vi "RW Current Limits.vi"(7 "Write?":bool, 8 "Low Lim 2":dbl[](array[numeric])=[-1.0, -1.0, -1.0, -1.0, -1.0, 3.5, 3.5, -1.0, -1.0, -1.0, -1.0, -1.0, -1.0, -1.0, -1.0, -1.0, -1.0, -1.0, -1.0, -1.0, -1.0, -1.0, -1.0, 22.0, -1.0, -1.0, -1.0, -1.0, -1.0, -1.0, -1.0, -1.0], 9 "Low Lim":dbl[](array[numeric])=[-1.0, -1.0, -1.0, -1.0, -1.0, 3.5, 3.5, -1.0, -1.0, -1.0, -1.0, -1.0, -1.0, -1.0, -1.0, -1.0, -1.0, -1.0, -1.0, -1.0, -1.0, -1.0, 22.0, -1.0, -1.0, -1.0, -1.0, -1.0, -1.0, -1.0, -1.0, -1.0], 10 "Up Lim":dbl[](array[numeric])=[50.0, 50.0, 50.0, 50.0, 50.0, 4.4, 4.4, 50.0, 50.0, 50.0, 50.0, 1.0, 1.0, 1.0, 50.0, 50.0, 50.0, 50.0, 50.0, 50.0, 27.0, 27.0, 27.0, 27.0, 27.0, 27.0, 27.0, 27.0, 1.0, 1.0, 1.0, 1.0], 11 "file path (dialog if empty)":path=path "c:/Data/Currents.csv") -> (1 "Low Lim 2 Out":dbl[](array[numeric])=[-1.0, -1.0, -1.0, -1.0, -1.0, 3.5, 3.5, -1.0, -1.0, -1.0, -1.0, -1.0, -1.0, -1.0, -1.0, -1.0, -1.0, -1.0, -1.0, -1.0, -1.0, -1.0, -1.0, 22.0, -1.0, -1.0, -1.0, -1.0, -1.0, -1.0, -1.0, -1.0], 2 "Low Lim Out":dbl[](array[numeric])=[-1.0, -1.0, -1.0, -1.0, -1.0, 3.5, 3.5, -1.0, -1.0, -1.0, -1.0, -1.0, -1.0, -1.0, -1.0, -1.0, -1.0, -1.0, -1.0, -1.0, -1.0, -1.0, 22.0, -1.0, -1.0, -1.0, -1.0, -1.0, -1.0, -1.0, -1.0, -1.0], 3 "Up Lim Out":dbl[](array[numeric])=[50.0, 50.0, 50.0, 50.0, 50.0, 4.4, 4.4, 50.0, 50.0, 50.0, 50.0, 1.0, 1.0, 1.0, 50.0, 50.0, 50.0, 50.0, 50.0, 50.0, 27.0, 27.0, 27.0, 27.0, 27.0, 27.0, 27.0, 27.0, 1.0, 1.0, 1.0, 1.0])   [LabVIEW 2012]
uses:
  <vilib>/Utility/file.llb/Read From Spreadsheet File (DBL).vi
  <vilib>/Utility/file.llb/Write To Spreadsheet File (DBL).vi
panel:
  out "all rows":dbl[][](array[numeric]) format="%0.3f"
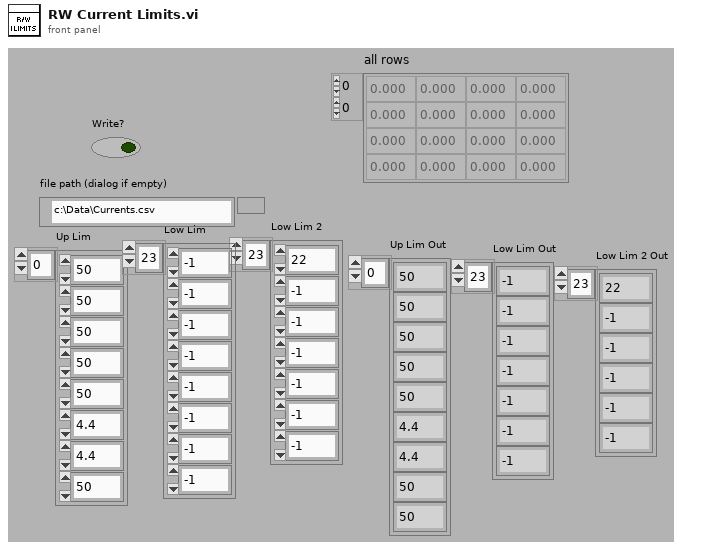
[diagram p1: front panel]
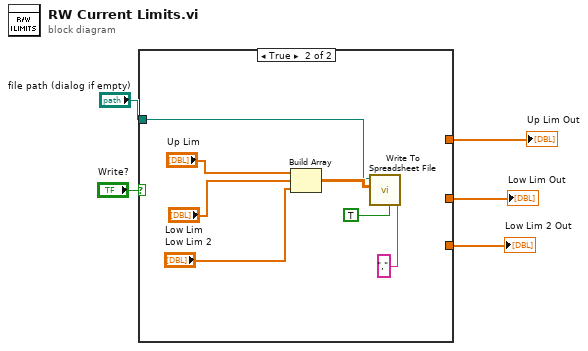
[diagram p0: block diagram]
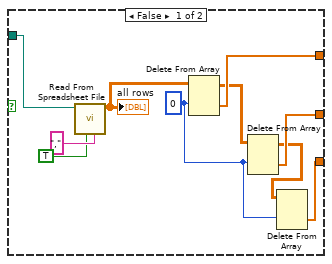
[diagram p2: hidden frame]
diagram:
  n1 = case shown="True" "Write?" {
    tunnel: "file path (dialog if empty)" -> [w14 w17]
    tunnel: [w12 _] -> w3
    tunnel: [w10 _] -> w2
    tunnel: [w7 _] -> w1
    frame False {
      w8 = 0 ("index (row)")
      n2 = call-poly <vilib>:"Read From Spreadsheet File.vi"("delimiter (\\t)"="," ("delimiter (\\t)"), "transpose (no:F)"=TRUE, "file path (dialog if empty)"=w14) -> ("all rows"=w13:dbl[][])  [unwired: 4 in, 4 out]
      "all rows" <- w13
      n3 = Delete From Array(array=w13, index (row)=w8) -> (deleted portion=w12:dbl[], array with subset deleted=w11:dbl[][])  [unwired: 2 in]
      n4 = Delete From Array(array=w11, index (row)=w8) -> (deleted portion=w10:dbl[], array with subset deleted=w9:dbl[][])  [unwired: 2 in]
      n5 = Delete From Array(array=w9, index (row)=w8) -> (deleted portion=w7:dbl[])  [unwired: 2 in, 1 out]
    }
    frame True {
      n6 = Build Array("Up Lim", "Low Lim", "Low Lim 2") -> (w19:dbl[][])
      n7 = call-poly <vilib>:"Write To Spreadsheet File.vi"("delimiter (\\t)"="," ("delimiter (\\t)"), "transpose? (no:F)"=TRUE, "2D data"=w19, "file path (dialog if empty)"=w17) -> ()  [unwired: 4 in, 1 out]
    }
  }
  "Up Lim Out" <- w3
  "Low Lim Out" <- w2
  "Low Lim 2 Out" <- w1
